vi "Q8381 CENTER.vi"(0 "VISA resource name":refnum<visa-resource-name>, 1 "Func":u16(ring) items=["CENTER", "PEAK", "CURSOR", "AUTO PKC"], 2 "Set value":dbl format="%.6f", 3 "unit/off/on":u16(ring) items=["um ", "nm", "OFF", "ON"], 4 "GPIB Address":u16=8 step=1) -> (5 "GPIB Status":bool)   [LabVIEW 2017]
doc: "func: 0: Center 1: Peak\n 2: Cursor 3: Auto PKC\nunit/off/on: 0: um 1: nm\n 2: off 3: on"
panel:
  out "Program code":string
  # "CENTER"
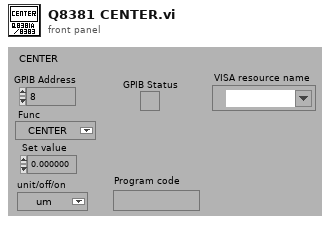
[diagram p1: front panel]
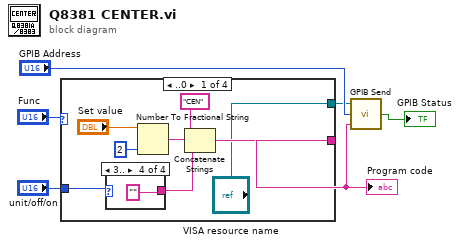
[diagram p0: block diagram]
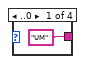
[diagram p2: hidden frame]
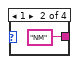
[diagram p3: hidden frame]
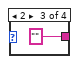
[diagram p4: hidden frame]
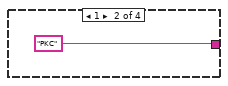
[diagram p5: hidden frame]
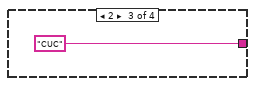
[diagram p6: hidden frame]
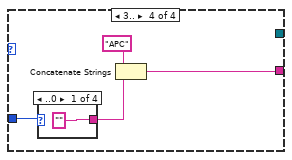
[diagram p7: hidden frame]
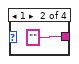
[diagram p8: hidden frame]
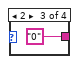
[diagram p9: hidden frame]
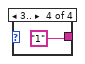
[diagram p10: hidden frame]
diagram:
  n1 = case shown="..0" "Func" {
    tunnel: [w9 "PKC" "CUC" w23] -> w4
    tunnel: "unit/off/on" -> [w8 _ _ w22]
    tunnel: ["VISA resource name" _ _ _] -> w2
    frame ..0 {
      n2 = case shown="3.." w8 {
        tunnel: ["UM" "NM" "" ""] -> w10
        frame ..0 {
        }
        frame 1 {
        }
        frame 2 {
        }
        frame 3.. {
        }
      }
      n3 = Number To Fractional String(number="Set value", precision (6)=2) -> (F-format string=w11:string)  [unwired: 2 in]
      n4 = Concatenate Strings("CEN", w11, w10) -> (w9:string)
    }
    frame 1 {
    }
    frame 2 {
    }
    frame 3.. {
      n5 = case shown="..0" w22 {
        tunnel: ["" "" "0" "1"] -> w21
        frame ..0 {
        }
        frame 1 {
        }
        frame 2 {
        }
        frame 3.. {
        }
      }
      n6 = Concatenate Strings("APC", w21) -> (w23:string)
    }
  }
  "Program code" <- w4
  n7 = call "GPIB Send.vi"("Command String"=w4, "Address"="GPIB Address", "VISA resource name"=w2) -> ("Error"=→"GPIB Status":bool)
